vi "increment_timepoint.vi"(8 "error in":errorcluster, 11 "EXPERIMENT SETTINGS IN":refnum<notifier>) -> (0 "error out":errorcluster, 3 "EXPERIMENT SETTINGS OUT":refnum<notifier>)   [LabVIEW 2013]
uses:
  type_defs/experiment_settings.ctl
  type_defs/experiment_states.ctl
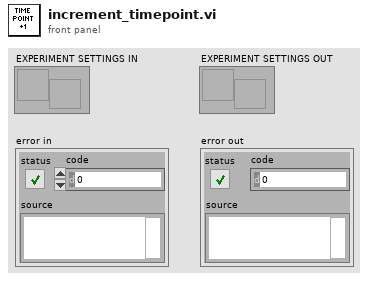
[diagram p1: front panel]
types:
  T1 = typedef "experiment_settings.ctl" = cluster{"fcs file byte offset":i64, "LED Device Handle Out":u32, "START TIME":timestamp, "CURRENT VALVE":u32, "SAMPLE #":i32, "FCS FILE PATH":path, "TIME POINT":i32, "STATE":T2, "TIME TILL SAMPLE":dbl, "DILUTION  TABLE":dbl[][]}
  T2 = typedef "experiment_states.ctl" = enum16{"OUTGROWTH", "INDUCTION", "EXPERIMENT"}
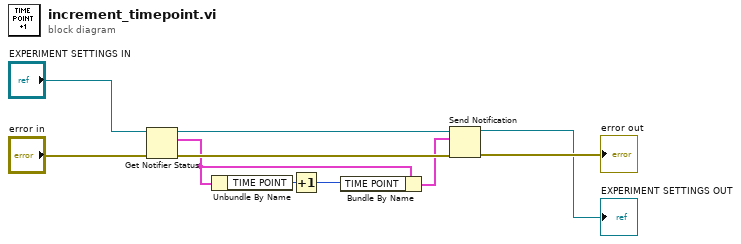
[diagram p0: block diagram]
diagram:
  n1 = Get Notifier Status(notifier="EXPERIMENT SETTINGS IN", error in (no error)="error in") -> (notifier out=w5:refnum<notifier>, current notification=w1:T1, error out=w10:errorcluster)  [unwired: 2 out]
  n2 = Unbundle By Name(w1) -> ("TIME POINT"=w3:i32)
  n3 = Increment(x=w3) -> (x+1=w4:i32)
  n4 = Bundle By Name(cluster=w1, "TIME POINT"=w4) -> (w7:T1)
  n5 = Send Notification(notification=w7, notifier=w5, error in (no error)=w10) -> (notifier out=→"EXPERIMENT SETTINGS OUT":refnum<notifier>, error out=→"error out":errorcluster)
